vi "Get Motor Label by Index.vi"(8 "error in (no error)":errorcluster, 10 "Index":i32, 11 "Motions in":refnum<class "Motions.lvclass">) -> (0 "error out":errorcluster, 1 "Index In Range?":bool, 2 "Label":string, 3 "Motions out":refnum<class "Motions.lvclass">)   [LabVIEW 2016, in "Hardware.lvlib" / "Motions.lvlib" / "Motions.lvclass"]
uses:
  <userlib>/Common Components/Hardware/Abstract System/Motions/Motions/Motions.lvclass
  <userlib>/Common Components/Hardware/Abstract System/Motions/Motions/Motions.lvclass/Motions.ctl
  <userlib>/Common Components/Hardware/Abstract Hardware/Hardware.lvclass/Hardware.ctl
  <userlib>/Common Components/Hardware/Abstract Hardware/Read Label.vi
  <userlib>/Common Components/Hardware/Motor/Motor/Motor.lvclass
  C:/Program Files (x86)/National Instruments/LabVIEW 2016/user.lib/Common Components/Hardware/Abstract Hardware/Hardware.lvclass
  <vilib>/Utility/error.llb/Error Cluster From Error Code.vi
  <vilib>/ErrorRing/Error Ring.xnode
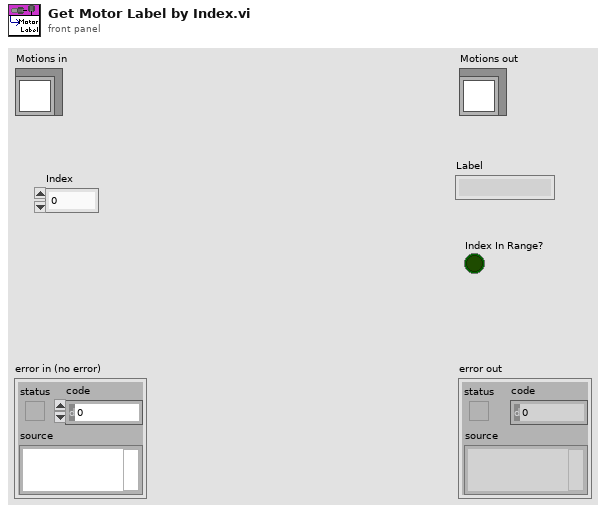
[diagram p1: front panel]
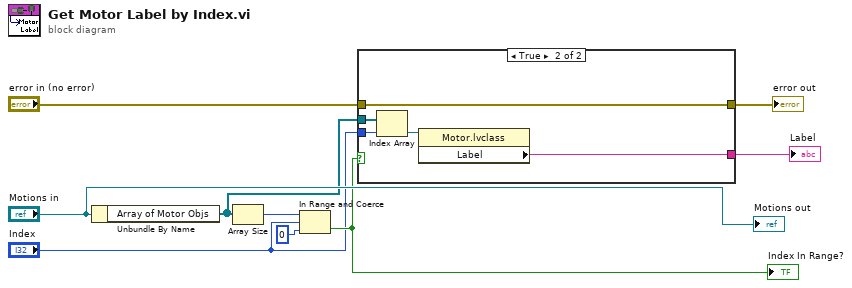
[diagram p0: block diagram]
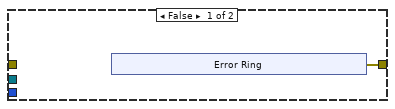
[diagram p2: hidden frame]
diagram:
  n1 = Unbundle By Name("Motions in") -> ("Array of Motor Objs"=w5:refnum<class "Motor.lvclass">[])
  n2 = Array Size(array=w5) -> (size(s)=w7:i32)
  n3 = In Range and Coerce(upper limit=w7, x="Index", lower limit=0) -> (In Range?=w6:bool)  [unwired: 1 out]
  "Index In Range?" <- w6
  n4 = case shown="True" w6 {
    tunnel: w5 -> [_ w19]
    tunnel: "Index" -> [_ w18]
    tunnel: [_ w16] -> w3
    tunnel: "error in (no error)" -> [_ w15]
    tunnel: [w10 w15] -> w1
    frame False {
      n5 = xnode "Error Ring"() -> ("error out"=w10:errorcluster)
    }
    frame True {
      n6 = Index Array(array=w19, index=w18) -> (element=w17:refnum<class "Motor.lvclass">)
      n7 = property class="Motor.lvclass"(reference=w17) -> ("Label"=w16:string)  [unwired: 1 in, 2 out]
    }
  }
  "error out" <- w1
  "Label" <- w3
  "Motions out" <- "Motions in"
